vi "Add Aliases.vi"(7 "Runtime Alias Folder Name":string, 8 "Error in":errorcluster, 9 "Alias Names":string[](array[string]), 10 "Referenced Channels":string[](array[string]), 11 "Runtime Configuration Ref in":refnum<k24>) -> (0 "Error out":errorcluster, 3 "Runtime Configuration Ref out":refnum<k24>)   [LabVIEW 2026, in "NIVS Runtime Configuration File Scripting API.lvlib"]
uses:
  NIVS Runtime Configuration File Scripting API.lvlib
  NationalInstruments.VeriStand.SystemDefinitionAPI
  <vilib>/NI/NI VeriStand Runtime Configuration File API/Runtime Configuration File API.lvlib
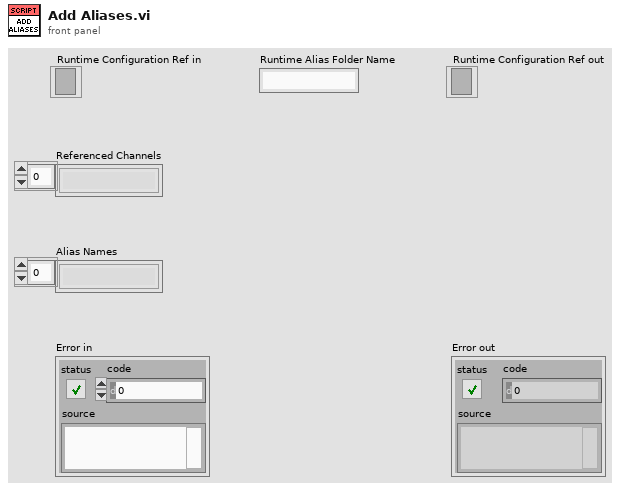
[diagram p1: front panel]
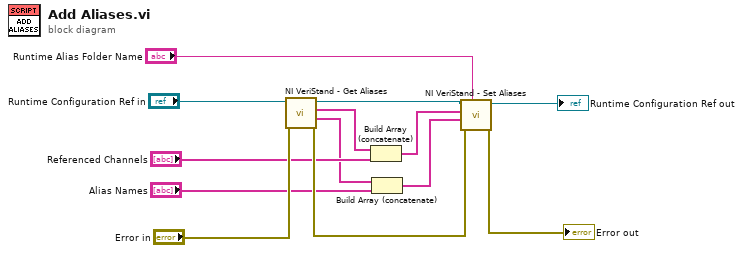
[diagram p0: block diagram]
diagram:
  n1 = call <vilib>:"NI VeriStand - Get Aliases.vi"("Error in"="Error in", "Runtime Configuration Ref in"="Runtime Configuration Ref in") -> ("Error out"=w12:errorcluster, "Alias Names"=w6:string[], "Referenced Channels"=w9:string[], "Runtime Configuration Ref out"=w3:refnum<k24>)  [unwired: 4 in, 2 out]
  n2 = Build Array (concatenate)(w9, "Referenced Channels") -> (w7:string[])
  n3 = Build Array (concatenate)(w6, "Alias Names") -> (w4:string[])
  n4 = call <vilib>:"NI VeriStand - Set Aliases.vi"("Runtime Alias Folder Name"="Runtime Alias Folder Name", "Error in"=w12, "Alias Names"=w4, "Referenced Channels"=w7, "Runtime Configuration Ref in"=w3) -> ("Error out"=→"Error out":errorcluster, "Runtime Configuration Ref out"=→"Runtime Configuration Ref out":refnum<k24>)  [unwired: 4 in, 1 out]
